vi "ROI group-Group naming handler.vi"(9 "POI group info cluster in":T1 {"Group region specifier cluster"."Contours"."Type" items=["No Selection", "Point", "Line", "Rectangle", "Oval", "Polygon", "Freehand Region", "Annulus", "Unused2", "Unused3", "Broken Line", "Freehand Line", "Rotated Rectangle"]}, 11 "New group (F)":bool) -> (1 "Cancelled?":bool, 3 "Group name":string)   [LabVIEW 2020]
uses:
  ROI Selection Interface/ROI group info cluster.ctl
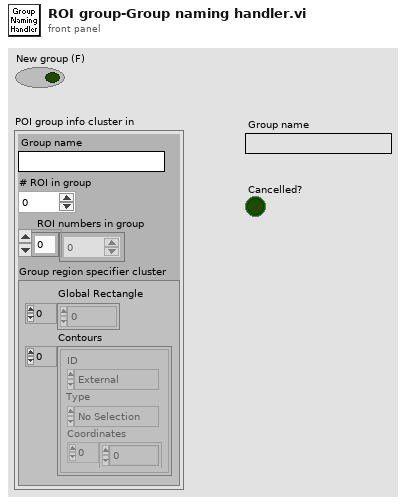
[diagram p1: front panel]
types:
  T1 = typedef "ROI group info cluster.ctl" = cluster{"Group name":string, "# ROI in group":i32, "ROI numbers in group":i32[], "Group region specifier cluster":T2}
  T2 = typedef "ROI Descriptor" = cluster{"Global Rectangle":i32[], "Contours":cluster{"ID":enum32{"External", "Internal"}, "Type":u32, "Coordinates":i32[]}[]}
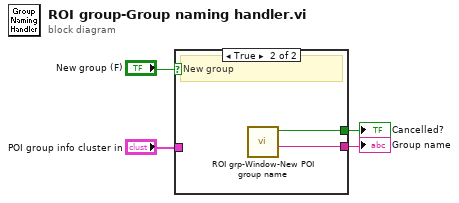
[diagram p0: block diagram]
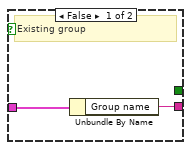
[diagram p2: hidden frame]
diagram:
  n1 = case shown="True" "New group (F)" {
    tunnel: "POI group info cluster in" -> [w6 _]
    tunnel: [w5 w7] -> w2
    tunnel: [_ w8] -> w1
    frame False {
      # "Existing group"
      n2 = Unbundle By Name(w6) -> ("Group name"=w5:string)
    }
    frame True {
      # "New group"
      n3 = call "ROI grp-Window-New POI group name.vi"() -> ("Group Name out"=w7:string, "Cancelled?"=w8:bool)  [unwired: 10 in]
    }
  }
  "Group name" <- w2
  "Cancelled?" <- w1
